vi "File HDF5 Open.vi"(8 "error in (no error)":errorcluster, 11 "File Path":path) -> (0 "error out":errorcluster, 3 "HDF IDs out":T1)   [LabVIEW 2011]
uses:
  Types Definitions/Type HDF IDs.ctl
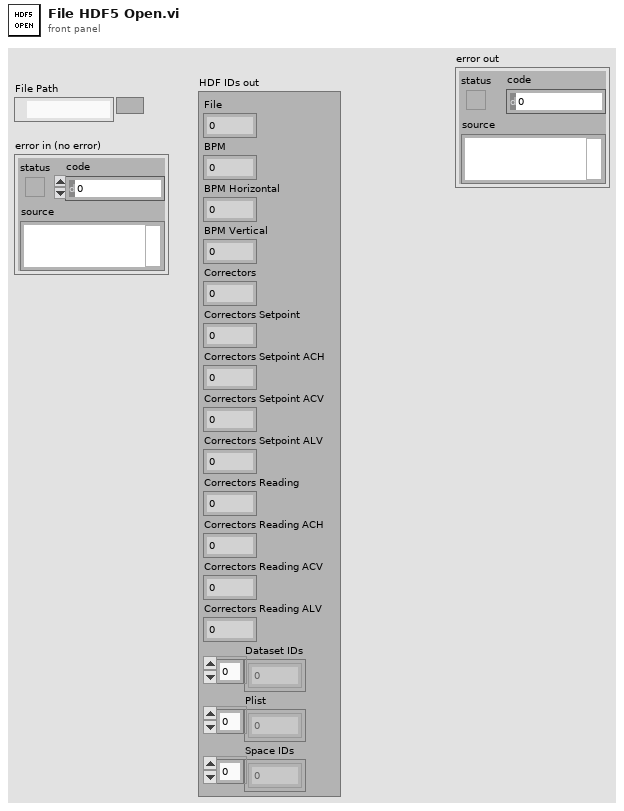
[diagram p1: front panel]
types:
  T1 = typedef "Type HDF IDs.ctl" = cluster{"File":i32, "BPM":i32, "BPM Horizontal":i32, "BPM Vertical":i32, "Correctors":i32, "Correctors Setpoint":i32, "Correctors Setpoint ACH":i32, "Correctors Setpoint ACV":i32, "Correctors Setpoint ALV":i32, "Correctors Reading":i32, "Correctors Reading ACH":i32, "Correctors Reading ACV":i32, "Correctors Reading ALV":i32, "Dataset IDs":i32[], "Plist":i32[], "Space IDs":i32[]}
  T2 = enum16{"open", "open or create", "create or replace", "create", "open (read only)"}
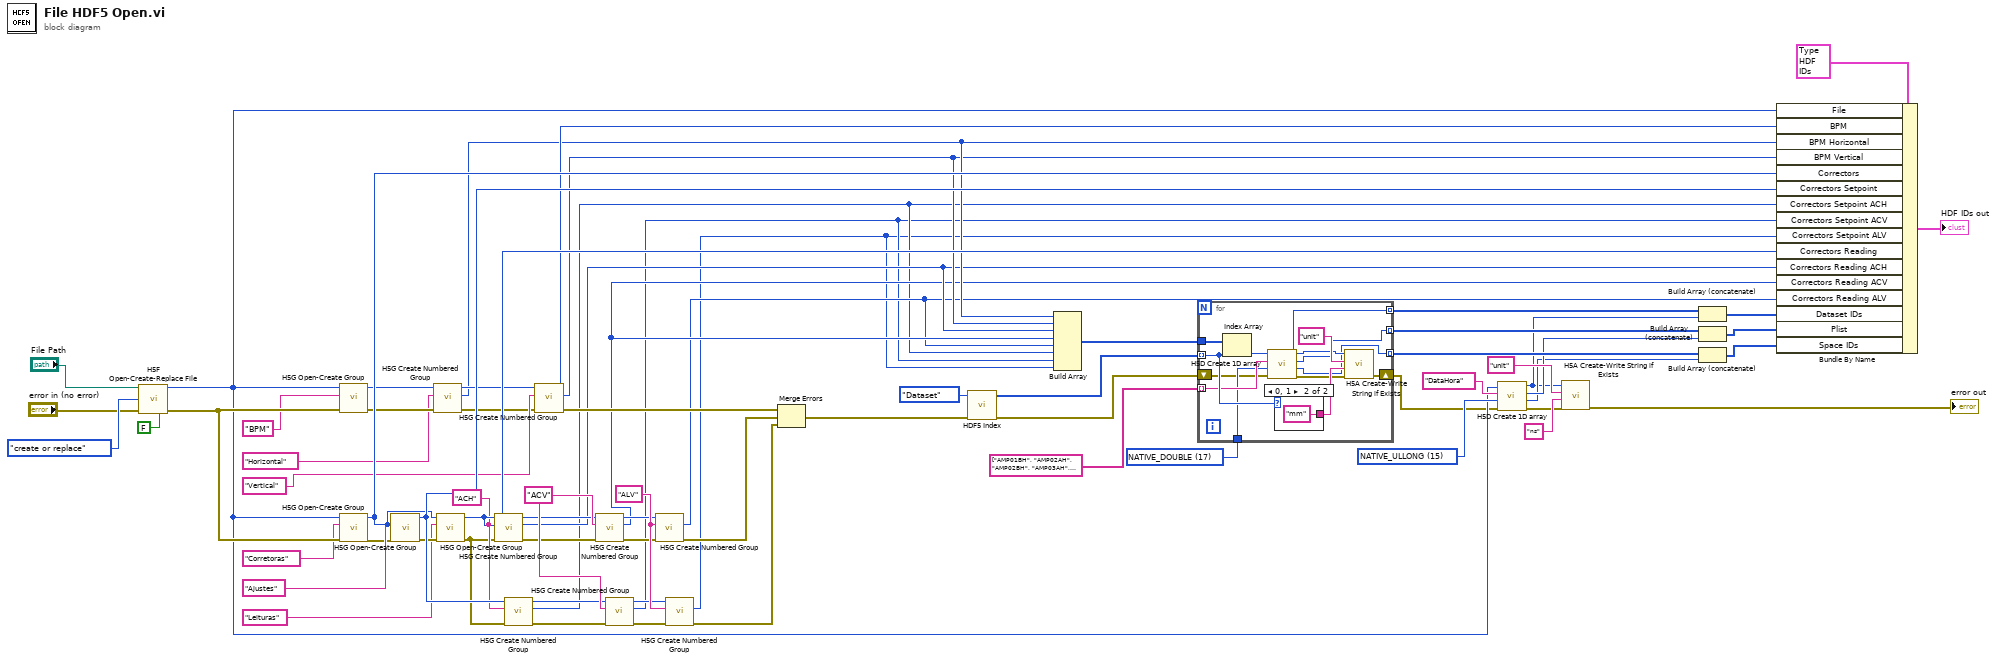
[diagram p0: block diagram]
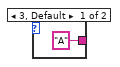
[diagram p2: hidden frame]
diagram:
  w26 = 15 items=["None", "IEEE_F32BE", "IEEE_F32LE", "IEEE_F64BE", "IEEE_F64LE", "NATIVE_CHAR", "NATIVE_SCHAR", "NATIVE_UCHAR", "NATIVE_SHORT", "NATIVE_USHORT", "NATIVE_INT", "NATIVE_UINT", "NATIVE_LONG", "NATIVE_ULONG", "NATIVE_LLONG", "NATIVE_ULLONG", "NATIVE_FLOAT", "NATIVE_DOUBLE", "NATIVE_LDOUBLE", "NATIVE_B8", "NATIVE_B16", "NATIVE_B32", "NATIVE_B64", "NATIVE_OPAQUE", "NATIVE_HADDR", "NATIVE_HSIZE", "NATIVE_HSSIZE", "NATIVE_HERR", "NATIVE_HBOOL", "STD_U8LE", "STD_U8BE", "STD_U16LE", "STD_U16BE", "STD_U32LE", "STD_U32BE", "STD_U64LE", "STD_U64BE", "STD_B8LE", "STD_B8BE", "STD_B16LE", "STD_B16BE", "STD_B32LE", "STD_B32BE", "STD_B64LE", "STD_B64BE", "STD_REF_OBJ", "STD_REF_DSETREG", "C_S1", "STD_I8LE", "STD_I8BE", "STD_I16LE", "STD_I16BE", "STD_I32LE", "STD_I32BE", "STD_I64LE", "STD_I64BE", ""] ("defined type")
  w27 = 17 items=["None", "IEEE_F32BE", "IEEE_F32LE", "IEEE_F64BE", "IEEE_F64LE", "NATIVE_CHAR", "NATIVE_SCHAR", "NATIVE_UCHAR", "NATIVE_SHORT", "NATIVE_USHORT", "NATIVE_INT", "NATIVE_UINT", "NATIVE_LONG", "NATIVE_ULONG", "NATIVE_LLONG", "NATIVE_ULLONG", "NATIVE_FLOAT", "NATIVE_DOUBLE", "NATIVE_LDOUBLE", "NATIVE_B8", "NATIVE_B16", "NATIVE_B32", "NATIVE_B64", "NATIVE_OPAQUE", "NATIVE_HADDR", "NATIVE_HSIZE", "NATIVE_HSSIZE", "NATIVE_HERR", "NATIVE_HBOOL", "STD_U8LE", "STD_U8BE", "STD_U16LE", "STD_U16BE", "STD_U32LE", "STD_U32BE", "STD_U64LE", "STD_U64BE", "STD_B8LE", "STD_B8BE", "STD_B16LE", "STD_B16BE", "STD_B32LE", "STD_B32BE", "STD_B64LE", "STD_B64BE", "STD_REF_OBJ", "STD_REF_DSETREG", "C_S1", "STD_I8LE", "STD_I8BE", "STD_I16LE", "STD_I16BE", "STD_I32LE", "STD_I32BE", "STD_I64LE", "STD_I64BE", ""] ("defined type")
  w62 = "ALV" ("base group name")
  w61 = "ACV" ("base group name")
  w60 = "ACH"
  n1 = call <instrlib>:"H5F Open-Create-Replace File.vi"("file path"="File Path", "function (open:0)"=T2."create or replace", "error in (not an error)"="error in (no error)", "advisory dialog? (display:T)"=FALSE) -> ("file id"=w24:i32, "error out"=w64:errorcluster)  [unwired: 9 in, 1 out]
  n2 = call <instrlib>:"H5G Open-Create Group.vi"("error in (no error)"=w64, "name"="BPM" ("base group name"), "loc_id"=w24) -> ("error out"=w45:errorcluster, "group_id"=w44:i32)  [unwired: 7 in]
  n3 = call <instrlib>:"H5G Open-Create Group.vi"("error in (no error)"=w64, "name"="Corretoras", "loc_id"=w24) -> ("error out"=w48:errorcluster, "group_id"=w67:i32)  [unwired: 7 in]
  n4 = call <instrlib>:"H5G Open-Create Group.vi"("error in (no error)"=w48, "name"="Ajustes", "loc_id"=w67) -> ("error out"=w55:errorcluster, "group_id"=w68:i32)  [unwired: 7 in]
  n5 = call <instrlib>:"H5G Create Numbered Group.vi"("error in (no error)"=w45, "base group name"="Horizontal", "loc_id"=w44) -> ("error out"=w41:errorcluster, "group_id"=w34:i32, "dup loc_id"=w43:i32)  [unwired: 4 in, 2 out]
  n6 = call <instrlib>:"H5G Open-Create Group.vi"("error in (no error)"=w55, "name"="Leituras", "loc_id"=w67) -> ("error out"=w56:errorcluster, "group_id"=w69:i32)  [unwired: 7 in]
  n7 = call <instrlib>:"H5G Create Numbered Group.vi"("error in (no error)"=w56, "base group name"=w60, "loc_id"=w69) -> ("error out"=w47:errorcluster, "group_id"=w10:i32, "dup loc_id"=w46:i32)  [unwired: 4 in, 2 out]
  n8 = call <instrlib>:"H5G Create Numbered Group.vi"("error in (no error)"=w56, "base group name"=w60, "loc_id"=w68) -> ("error out"=w54:errorcluster, "group_id"=w7:i32, "dup loc_id"=w11:i32)  [unwired: 4 in, 2 out]
  n9 = call <instrlib>:"H5G Create Numbered Group.vi"("error in (no error)"=w41, "base group name"="Vertical", "loc_id"=w43) -> ("error out"=w57:errorcluster, "group_id"=w33:i32, "dup loc_id"=w66:i32)  [unwired: 4 in, 2 out]
  n10 = call <instrlib>:"H5G Create Numbered Group.vi"("error in (no error)"=w47, "base group name"=w61, "loc_id"=w46) -> ("error out"=w51:errorcluster, "group_id"=w9:i32, "dup loc_id"=w12:i32)  [unwired: 4 in, 2 out]
  n11 = call <instrlib>:"H5G Create Numbered Group.vi"("error in (no error)"=w54, "base group name"=w61, "loc_id"=w11) -> ("error out"=w52:errorcluster, "group_id"=w6:i32, "dup loc_id"=w53:i32)  [unwired: 4 in, 2 out]
  n12 = call <instrlib>:"H5G Create Numbered Group.vi"("error in (no error)"=w51, "base group name"=w62, "loc_id"=w12) -> ("error out"=w58:errorcluster, "group_id"=w8:i32)  [unwired: 4 in, 3 out]
  n13 = call <instrlib>:"H5G Create Numbered Group.vi"("error in (no error)"=w52, "base group name"=w62, "loc_id"=w53) -> ("error out"=w59:errorcluster, "group_id"=w5:i32)  [unwired: 4 in, 3 out]
  n14 = Merge Errors(w57, w58, w59) -> (w28:errorcluster)
  n15 = call "HDF5 Index.vi"("error in (no error)"=w28, "Mapping Type"=enum16{"Dataset", "Variables"}."Dataset") -> ("error out"=w14:errorcluster, "Mapping out"=w35:i32[])  [unwired: 8 in]
  n16 = Build Array(w34, w33, w10, w9, w8, w7, w6, w5) -> (w32:i32[])
  n17 = for {
    tunnel: w32 -> [w82]
    tunnel: string[] ["AMP01BH", "AMP02AH", "AMP02BH", "AMP03AH", "AMP03BH", "AMP03CH", "AMP04AH", "AMP04BH", "AMP05AH", "AMP05BH", "AMP06AH", "AMP06BH", "AMP07AH", "AMP07BH", "AMP08AH", "AMP08BH", "AMP09AH", "AMP09BH", "AMP10AH", "AMP10BH", "AMU11AH", "AMU11BH", "AMP12AH", "AMP12BH", "AMP01AH", "AMP01BV", "AMP02AV", "AMP02BV", "AMP03AV", "AMP03BV", "AMP03CV", "AMP04AV", "AMP04BV", "AMP05AV", "AMP05BV", "AMP06AV", "AMP06BV", "AMP07AV", "AMP07BV", "AMP08AV", "AMP08BV", "AMP09AV", "AMP09BV", "AMP10AV", "AMP10BV", "AMU11AV", "AMU11BV", "AMP12AV", "AMP12BV", "AMP01AV", "ACH01B", "ACH02", "ACH03A", "ACH03B", "ACH04", "ACH05A", "ACH05B", "ACH06", "ACH07A", "ACH07B", "ACH08", "ACH09A", "ACH09B", "ACH10", "ACH11A", "ACH11B", "ACH12", "ACH01A", "ACV01B", "ACV03A", "ACV03B", "ACV05A", "ACV05B", "ACV07A", "ACV07B", "ACV09A", "ACV09B", "ACV11A", "ACV11B", "ACV01A", "ALV02A", "ALV02B", "ALV04A", "ALV04B", "ALV06A", "ALV06B", "ALV08A", "ALV08B", "ALV10A", "ALV10B", "ALV12A", "ALV12B", "ACH01B", "ACH02", "ACH03A", "ACH03B", "ACH04", "ACH05A", "ACH05B", "ACH06", "ACH07A", "ACH07B", "ACH08", "ACH09A", "ACH09B", "ACH10", "ACH11A", "ACH11B", "ACH12", "ACH01A", "ACV01B", "ACV03A", "ACV03B", "ACV05A", "ACV05B", "ACV07A", "ACV07B", "ACV09A", "ACV09B", "ACV11A", "ACV11B", "ACV01A", "ALV02A", "ALV02B", "ALV04A", "ALV04B", "ALV06A", "ALV06B", "ALV08A", "ALV08B", "ALV10A", "ALV10B", "ALV12A", "ALV12B"] ("appended array") -> [w78] mode=indexing
    tunnel: w35 -> [w80] mode=indexing
    tunnel: [w72] -> w19 mode=indexing
    tunnel: w27 -> [w77]
    tunnel: [w74] -> w20 mode=indexing
    tunnel: [w75] -> w21 mode=indexing
    shift-right: [w73] -> w13
    shift-left: w14 -> [w71]
    n18 = Index Array(array=w82, index=w80) -> (element=w79:i32)
    n19 = call "H5D Create 1D array.vi"("error in (no error)"=w71, "defined type"=w77, "name"=w78, "loc_id"=w79) -> ("error out"=w76:errorcluster, "space_id"=w72:i32, "plist out"=w74:i32, "dataset_id"=w75:i32)  [unwired: 4 in]
    n20 = case shown="0, 1" w80 {
      tunnel: ["A" ("value") "mm" ("value")] -> w81
      frame 3, Default {
      }
      frame 0, 1 {
      }
    }
    n21 = call <instrlib>:"H5A Create-Write String if Exists.vi"("error in (no error)"=w76, "value"=w81, "name"="unit", "loc_id"=w75) -> ("error out"=w73:errorcluster)  [unwired: 6 in, 1 out]
  }
  n22 = call "H5D Create 1D array.vi"("error in (no error)"=w13, "defined type"=w26, "name"="DataHora" ("Name"), "loc_id"=w24) -> ("error out"=w23:errorcluster, "space_id"=w17:i32, "plist out"=w18:i32, "dataset_id"=w2:i32)  [unwired: 4 in]
  n23 = call <instrlib>:"H5A Create-Write String if Exists.vi"("error in (no error)"=w23, "value"="ns" ("Unit"), "name"="unit", "loc_id"=w2) -> ("error out"=→"error out":errorcluster)  [unwired: 6 in, 1 out]
  n24 = Build Array (concatenate)(w21, w2) -> (w22:i32[])
  n25 = Build Array (concatenate)(w20, w18) -> (w16:i32[])
  n26 = Build Array (concatenate)(w19, w17) -> (w15:i32[])
  n27 = Bundle By Name(cluster=T1 {"File"=0, "BPM"=0, "BPM Horizontal"=0, "BPM Vertical"=0, "Correctors"=0, "Correctors Setpoint"=0, "Correctors Setpoint ACH"=0, "Correctors Setpoint ACV"=0, "Correctors Setpoint ALV"=0, "Correctors Reading"=0, "Correctors Reading ACH"=0, "Correctors Reading ACV"=0, "Correctors Reading ALV"=0, "Dataset IDs"=[], "Plist"=[], "Space IDs"=[]} ("HDF IDs"), "File"=w24, "BPM"=w66, "BPM Horizontal"=w34, "BPM Vertical"=w33, "Correctors"=w67, "Correctors Setpoint"=w68, "Correctors Setpoint ACH"=w7, "Correctors Setpoint ACV"=w6, "Correctors Setpoint ALV"=w5, "Correctors Reading"=w69, "Correctors Reading ACH"=w10, "Correctors Reading ACV"=w9, "Correctors Reading ALV"=w8, "Dataset IDs"=w22, "Plist"=w16, "Space IDs"=w15) -> (→"HDF IDs out":T1)
